vi "xps_panel_delete_user_events.vi"(8 "error in (no error)":errorcluster, 11 "newport_xps_panel in":refnum<class "newport_xps_panel.lvclass">) -> (0 "error out":errorcluster, 3 "newport_xps_panel out":refnum<class "newport_xps_panel.lvclass">)   [LabVIEW 2015, in "newport_xps_panel.lvclass"]
uses:
  newport_xps_panel.lvclass
  newport_xps_panel.lvclass/newport_xps_panel.ctl
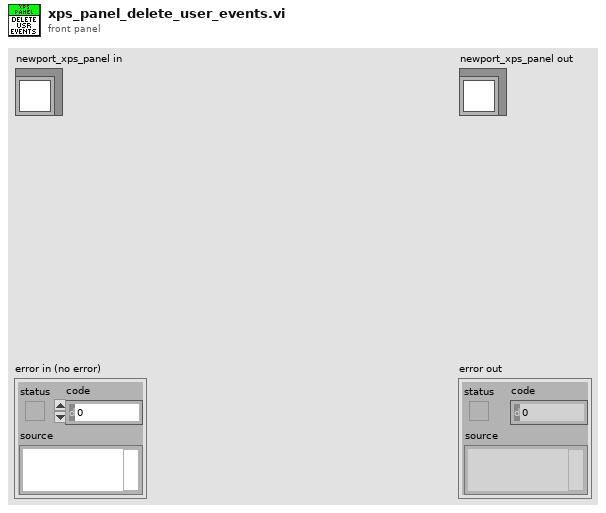
[diagram p1: front panel]
types:
  T1 = typedef "xps_user_events.ctl" = cluster{"xps_position":refnum<user-event>, "abort_move":refnum<user-event>, "update_xps_status":refnum<user-event>, "retrieve_trajectories":refnum<user-event>, "set_available_stages":refnum<user-event>}
  T2 = typedef "event_references.ctl" = cluster{"update_position":refnum<event-registration>, "abort_move":refnum<event-registration>, "update_xps_status":refnum<event-registration>, "retrieve_trajectories":refnum<event-registration>, "set_available_stages":refnum<event-registration>}
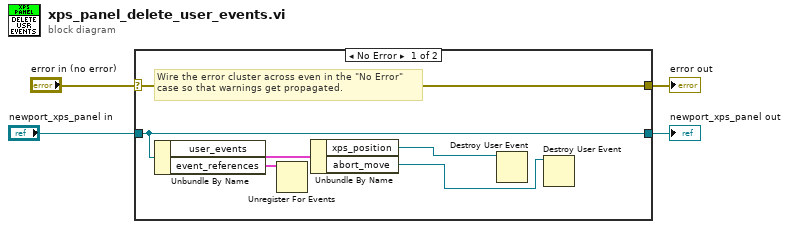
[diagram p0: block diagram]
diagram:
  n1 = case shown="No Error" "error in (no error)" {
    selector: "error in (no error)" -> [w10 w12]
    tunnel: [w10 w12] -> w3
    tunnel: [w7 w11] -> w1
    tunnel: "newport_xps_panel in" -> [w7 w11]
    frame No Error {
      # "Wire the error cluster across even in the \"No Error\"\ncase so that warnings get propagated."
      n2 = Unbundle By Name(w7) -> ("user_events"=w9:T1, "event_references"=w6:T2)
      n3 = Unregister For Events(event registration refnum=w6) -> ()  [unwired: 1 in, 1 out]
      n4 = Unbundle By Name(w9) -> ("xps_position"=w8:refnum<user-event>, "abort_move"=w5:refnum<user-event>)
      n5 = Destroy User Event(user event=w8) -> ()  [unwired: 1 in, 1 out]
      n6 = Destroy User Event(user event=w5) -> ()  [unwired: 1 in, 1 out]
    }
    frame Error {
    }
  }
  "error out" <- w3
  "newport_xps_panel out" <- w1
